vi "Teleop.vi"(10 "Match Info":T1={"Autonomous Elapsed Seconds"=0.0, "TeleOp Elapsed Seconds"=0.0, "Disabled Elapsed Seconds"=0.0, "Visited Autonomous"=FALSE, "Visited TeleOp"=FALSE, "Visited Disabled"=FALSE, "Autonomous Settings"={"Autonomous Style"=enum."Independent", "VI Refnum"=refnum}}, 11 "Call Context":T2) -> ()   [LabVIEW 2013]
doc: "This VI is called for each TeleOp packet received from the DS where the robot is not disabled. It is often used to read from the joysticks and update I/O or to update setpoints for timed control loops. It should complete and return within 20 milliseconds or it may miss DS packets."
uses:
  <vilib>/Rock Robotics/WPI/DriverStation/WPI_DriverStationDerivedRobotMode.ctl
  <vilib>/Rock Robotics/WPI/DriverStation/WPI_DriverStationMatch Info.ctl
  <vilib>/Rock Robotics/WPI/Solenoid/WPI_SolenoidValue.ctl
  Robot Global Data.vi
  <vilib>/Rock Robotics/WPI/Joystick/WPI_JoystickGetSetRefNum.vi
panel:
  in  "Xbox Controller?":bool
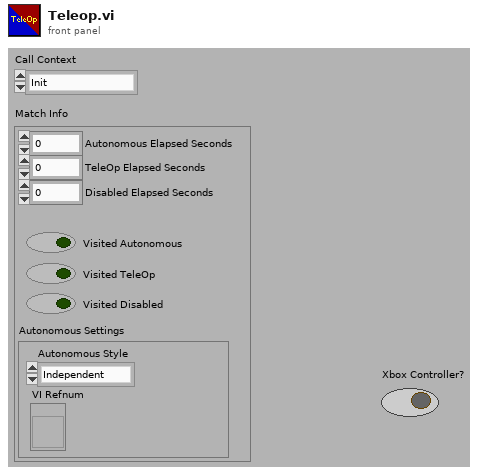
[diagram p1: front panel]
types:
  T1 = typedef "WPI_DriverStationMatch Info.ctl" = cluster{"Autonomous Elapsed Seconds":dbl, "TeleOp Elapsed Seconds":dbl, "Disabled Elapsed Seconds":dbl, "Visited Autonomous":bool, "Visited TeleOp":bool, "Visited Disabled":bool, "Autonomous Settings":cluster{"Autonomous Style":enum16{"Iterative", "Independent"}, "VI Refnum":refnum<vi>}}
  T2 = typedef "WPI_DriverStationDerivedRobotMode.ctl" = enum16{"Init", "Execute", "Stop"}
  T3 = typedef "WPI_SolenoidValue.ctl" = enum16{"Off", "On", "Forward", "Reverse"}
  T4 = typedef "WPI_ServoDeviceRef.ctl" = cluster{"DeviceStatus":errorcluster, "Digital Module":T5, "PWM Channel":T6, "DeadBand":T7}
  T5 = typedef "FPGA_TypedefDigitalModule.ctl" = enum16{"Digital Module 1", "Digital Module 2"}
  T6 = typedef "FPGA_DIOPWMChannel.ctl" = enum8{"PWM 1", "PWM 2", "PWM 3", "PWM 4", "PWM 5", "PWM 6", "PWM 7", "PWM 8", "PWM 9", "PWM 10", "Invalid"}
  T7 = typedef "WPI_PWMDeadband.ctl" = cluster{"Name":string, "maxPositivePwm":i32, "minPositivePwm":i32, "centerPwm":i32, "maxNegativePwm":i32, "minNegativePwm":i32, "angularRange":u16}
  T8 = typedef "WPI_JoystickDevRef.ctl" = cluster{"Device":T9}
  T9 = typedef "WPI_JoystickDeviceEnum.ctl" = enum16{"USB 1", "USB 2", "USB 3", "USB 4", "Kinect 1", "Kinect 2"}
  T10 = typedef "WPI_JoystickButtonState.ctl" = cluster{"Button 1":bool, "Button 2":bool, "Button 3":bool, "Button 4":bool, "Button 5":bool, "Button 6":bool, "Button 7":bool, "Button 8":bool, "Button 9":bool, "Button 10":bool, "Button 11":bool, "Button 12":bool}
  T11 = cluster{"axis 1 (x)":dbl, "axis 2 (y)":dbl, "axis 3 (throttle)":dbl, "axis 4":dbl, "axis 5":dbl, "axis 6":dbl}
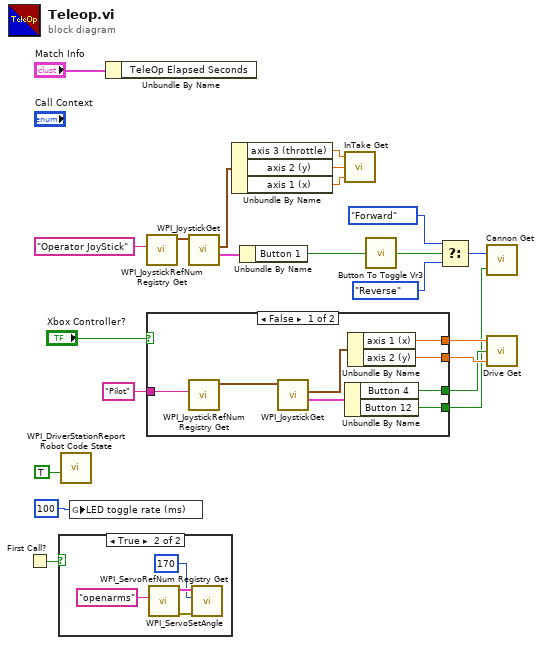
[diagram p0: block diagram]
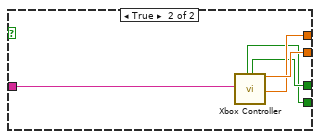
[diagram p3: hidden frame]
diagram:
  n1 = First Call?() -> (First Call?: T/F=w10:bool)
  n2 = case shown="True" w10 {
    frame False {
    }
    frame True {
      n3 = call <vilib>:"WPI_ServoRefNum Registry Get.vi"("refnum name"="openarms") -> ("error out"=w26:errorcluster, "ServoDeviceRef"=w25:T4)  [unwired: 9 in]
      n4 = call <vilib>:"WPI_ServoSetAngle.vi"("error in (no error)"=w26, "Angle"=170, "ServoDeviceRef"=w25) -> ()  [unwired: 7 in, 2 out]
    }
  }
  n5 = call <vilib>:"WPI_DriverStationReport Robot Code State.vi"("TeleOp"=TRUE ("Autonomous")) -> ()  [unwired: 10 in, 1 out]
  n6 = global write "Robot Global Data.vi" "LED toggle rate (ms)"(u32 100 ("LED ms toggle rate")) -> ()
  n7 = Unbundle By Name("Match Info") -> ()  [unwired: 1 out]
  n8 = call <vilib>:"WPI_JoystickRefNum Registry Get.vi"("refnum name"="Operator JoyStick") -> ("JoystickDevRef"=w8:T8)  [unwired: 9 in, 1 out]
  n9 = case shown="False" "Xbox Controller?" {
    tunnel: "Pilot" ("refnum name") -> [w33 w39]
    tunnel: [w31 w38] -> w17
    tunnel: [w30 w37] -> w16
    tunnel: [w28 w36] -> w11
    tunnel: [w27 w35] -> w9
    frame False {
      n10 = call <vilib>:"WPI_JoystickRefNum Registry Get.vi"("refnum name"=w33) -> ("JoystickDevRef"=w34:T8)  [unwired: 9 in, 1 out]
      n11 = call <vilib>:"WPI_JoystickGet.vi"("JoystickDevRef"=w34) -> ("Buttons"=w29:T10, "Axes"=w32:T11)  [unwired: 4 in, 1 out]
      n12 = Unbundle By Name(w29) -> ("Button 4"=w28:bool, "Button 12"=w27:bool)
      n13 = Unbundle By Name(w32) -> ("axis 1 (x)"=w30:dbl, "axis 2 (y)"=w31:dbl)
    }
    frame True {
      n14 = call "Xbox Controller.vi"("Joystick Name"=w39) -> ("Left Button"=w35:bool, "Right Button"=w36:bool, "Left Stick Y"=w38:dbl, "Right Stick Y"=w37:dbl)  [unwired: 3 in, 12 out]
    }
  }
  n15 = call <vilib>:"WPI_JoystickGet.vi"("JoystickDevRef"=w8) -> ("Buttons"=w6:T10, "Axes"=w7:T11)  [unwired: 4 in, 1 out]
  n16 = Unbundle By Name(w7) -> ("axis 3 (throttle)"=w2:dbl, "axis 2 (y)"=w4:dbl, "axis 1 (x)"=w1:dbl)
  n17 = Unbundle By Name(w6) -> ("Button 1"=w3:bool)
  n18 = call "InTake Get.vi"("LowerClaw"=w1, "UpperClaw"=w4, "TakeBall"=w2) -> ()
  n19 = call "Button To Toggle Vr3.vi"("InValue"=w3) -> ("Result"=w14:bool)
  n20 = Select(t=WPI_SolenoidValue."Forward" ("Shoot!"), s=w14, f=WPI_SolenoidValue."Reverse" ("Shoot!")) -> (s? t:f=w12:T3)
  n21 = call "Cannon Get.vi"("Reset Gyro?"=w9, "Shoot!"=w12) -> ()  [unwired: 1 in]
  n22 = call "Drive Get.vi"("Y"=w17, "Slow Drive"=w11, "X"=w16) -> ()  [unwired: 1 in]
